vi "Read Raw Log.vi"(5 "Component ID":u8, 7 "FPGA Interface":refnum<class "FPGA Interface.lvclass">, 8 "error in (no error)":errorcluster, 10 "bmReadConfig":T1={"cmdRecordStart"=21632, "cmdRecordLength"=2024, "dataRecordStart"=21632, "dataRecordEnd"=21632} {"dataRecordEnd" format="%04x"; "dataRecordStart" format="%04x"; "cmdRecordStart" format="%04x"}, 11 "48-bit Timetag?":bool) -> (0 "error out":errorcluster, 3 "Raw Log":u16[](array[numeric]) format="%.0x")   [LabVIEW 2016, in "BCI-1553 API.lvlib" / "Bus Monitor.lvclass"]
doc: "Performs the specific reads from the IC to retrieve the entire bus monitor log for a given block of memory. It additionally performs some slight reformatting to the data blocks to get a more easily parsed raw data array."
uses:
  Bus Monitor.lvclass
  Dependencies/FPGA Interface/FPGA Interface.lvclass
  TypeDefs/Bus Monitor Message Type.ctl
  Dependencies/FPGA Interface/rolloverReadConfig.ctl
  TypeDefs/Bus Monitor Read Config.ctl
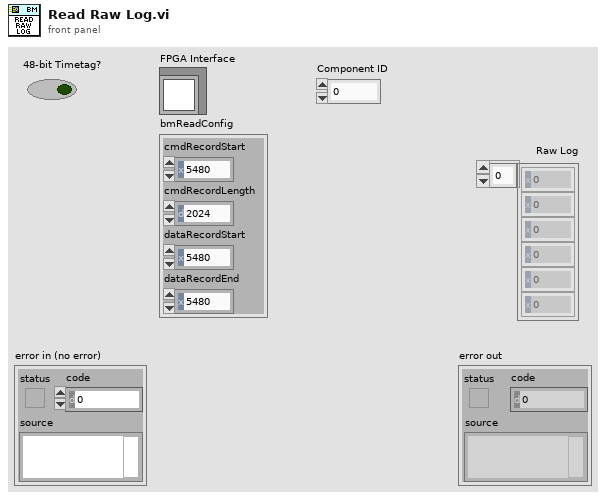
[diagram p1: front panel]
types:
  T1 = typedef "BCI-1553 API.lvlib/Bus Monitor.lvclass/Bus Monitor Read Config.ctl" = cluster{"cmdRecordStart":u16, "cmdRecordLength":u16, "dataRecordStart":u16, "dataRecordEnd":u16}
  T2 = typedef "BCI-1553 API.lvlib/Bus Monitor.lvclass/Bus Monitor Message Type.ctl" = enum16{"Transmit", "Receive", "RT-RT Message", "Mode Code Transmit", "Mode Code Receive", "NULL"}
  T3 = typedef "BCI-1553 API.lvlib/FPGA Interface.lvlib/FPGA Interface.lvclass/rolloverReadConfig.ctl" = cluster{"startAddr":u16, "lowerAddr":u16, "upperAddr":u16}
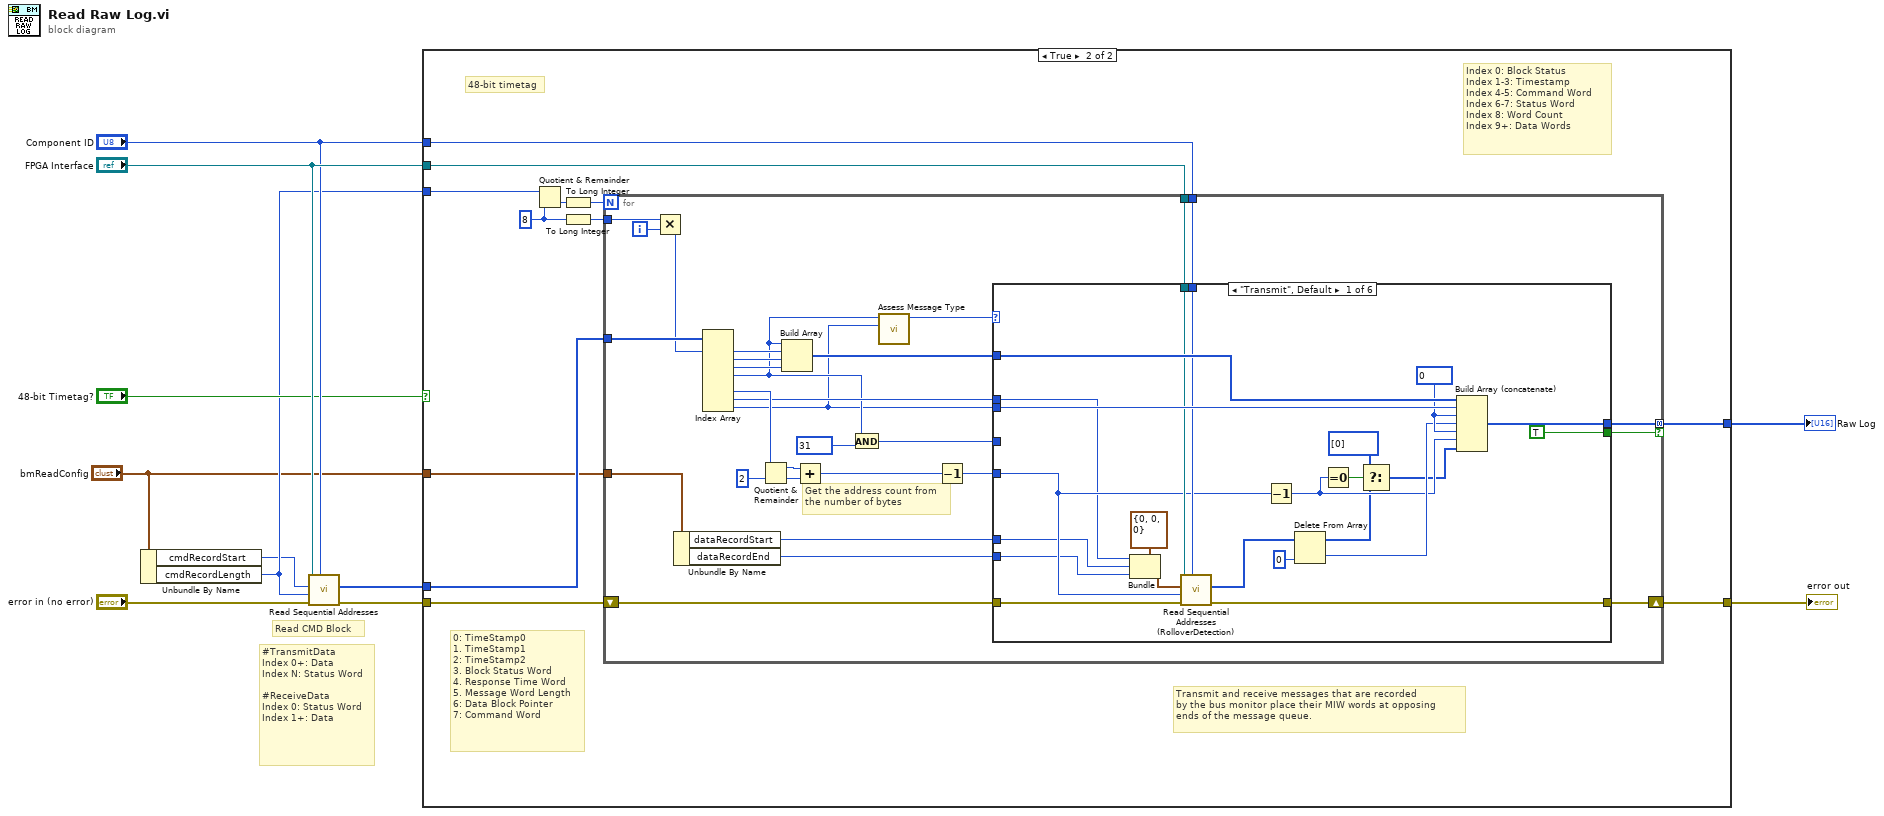
[diagram p0: block diagram]
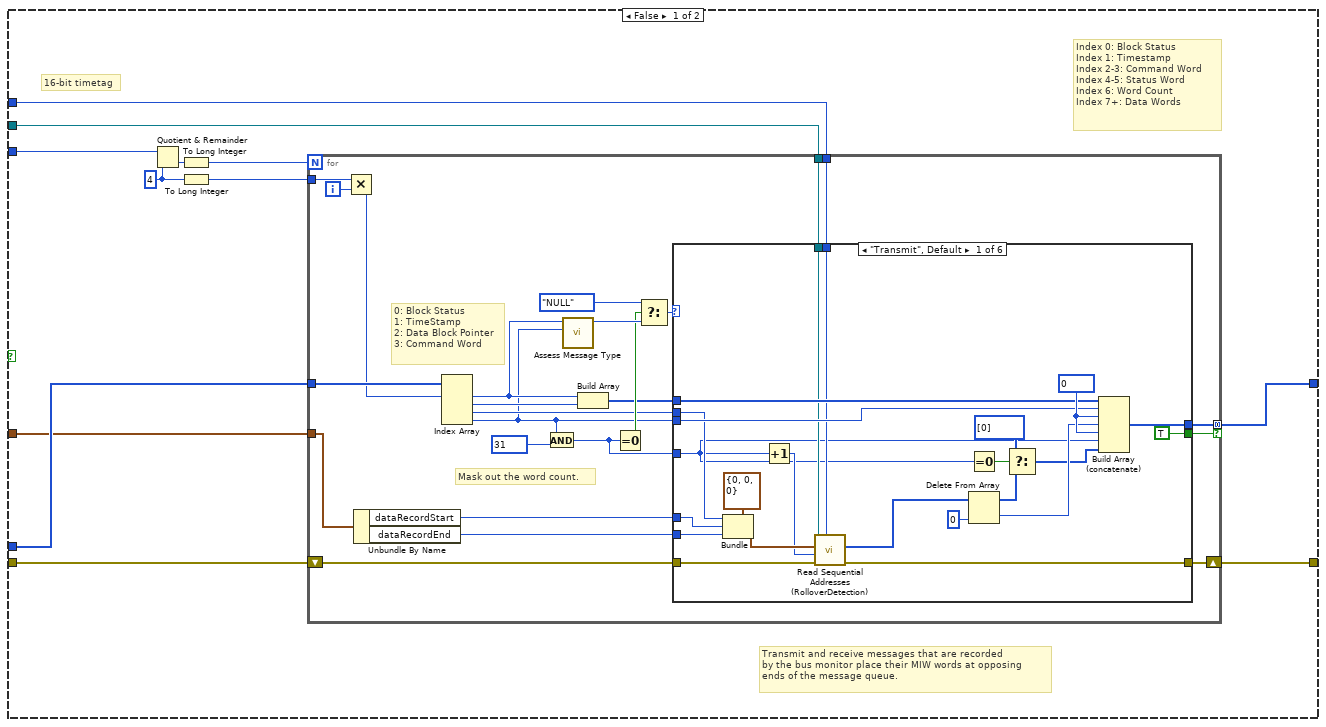
[diagram p2: hidden frame]
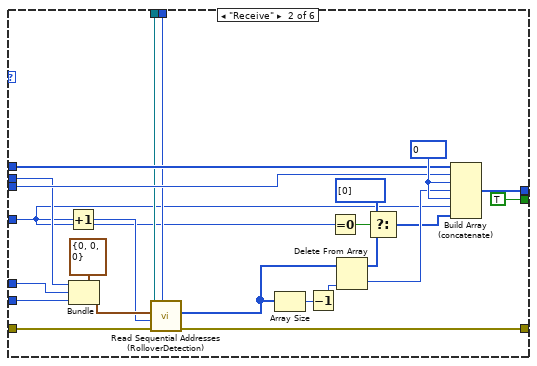
[diagram p3: hidden frame]
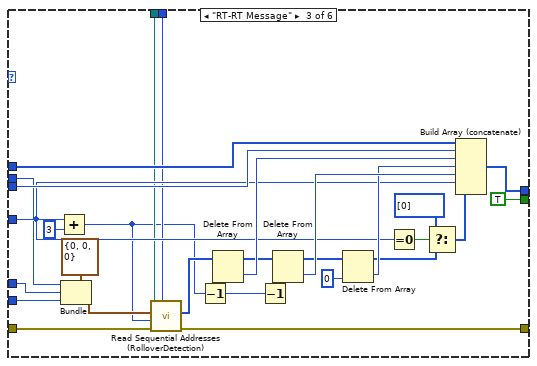
[diagram p4: hidden frame]
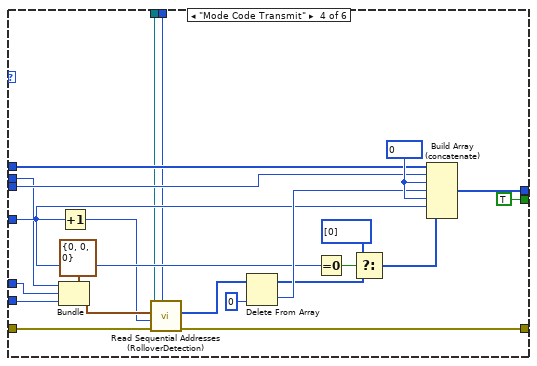
[diagram p5: hidden frame]
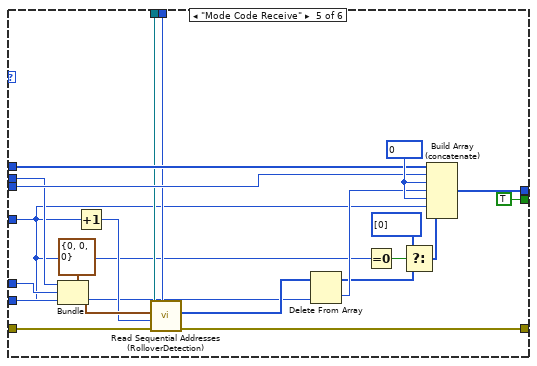
[diagram p6: hidden frame]
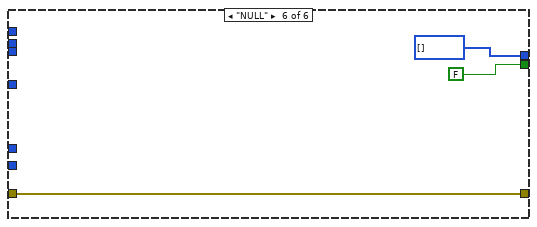
[diagram p7: hidden frame]
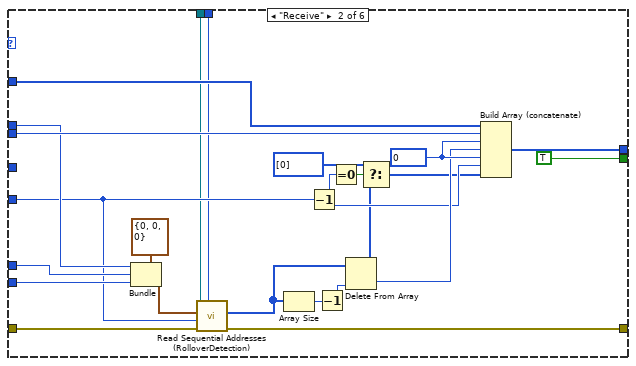
[diagram p8: hidden frame]
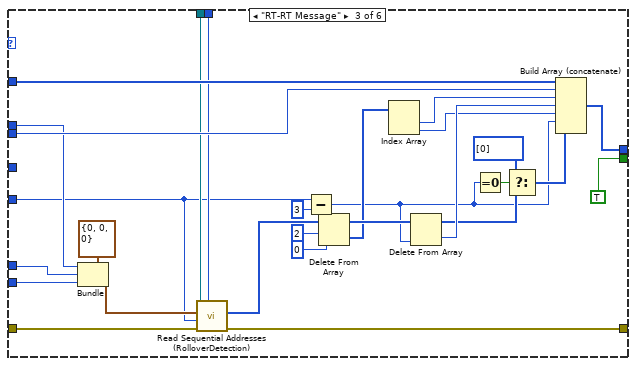
[diagram p9: hidden frame]
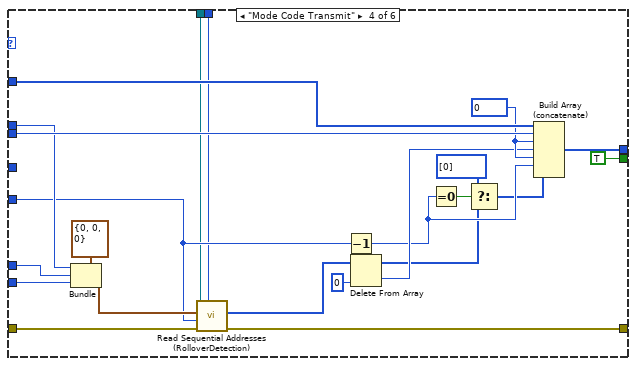
[diagram p10: hidden frame]
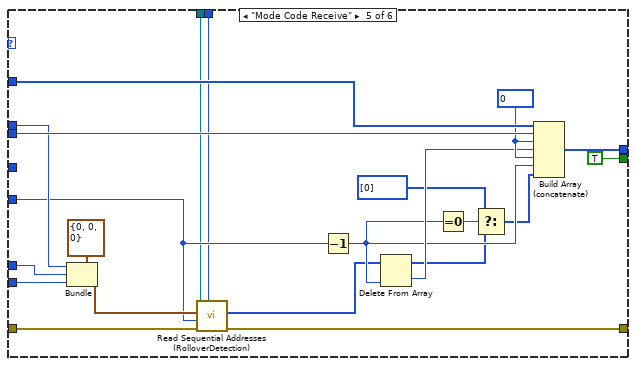
[diagram p11: hidden frame]
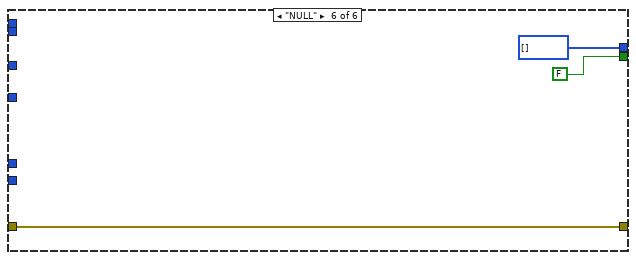
[diagram p12: hidden frame]
diagram:
  # "#TransmitData\nIndex 0+: Data\nIndex N: Status Word\n\n#ReceiveData\nIndex 0: Status Word\nIndex 1+: Data"
  # "Read CMD Block"
  n1 = Unbundle By Name("bmReadConfig") -> ("cmdRecordStart"=w2:u16, "cmdRecordLength"=w3:u16)
  n2 = call-dynamic "Read Sequential Addresses.vi"("Target IC (1-8)"="Component ID", "error in (no error)"="error in (no error)", "Addresses to Read"=w3, "Starting Address"=w2, "FPGA Interface in"="FPGA Interface") -> ("error out"=w11:errorcluster, "Data"=w10:u16[])  [unwired: 5 in]
  n3 = case shown="True" "48-bit Timetag?" {
    tunnel: w11 -> [w23 w183]
    tunnel: w10 -> [w22 w182]
    tunnel: [w18 w178] -> w8
    tunnel: "FPGA Interface" -> [w17 w177]
    tunnel: "Component ID" -> [w16 w176]
    tunnel: w3 -> [w15 w175]
    tunnel: [w14 w174] -> w5
    tunnel: "bmReadConfig" -> [w12 w172]
    frame False {
      w13 = u16 4 ("y")
      # "Index 0: Block Status\nIndex 1: Timestamp\nIndex 2-3: Command Word\nIndex 4-5: Status Word\nIndex 6: Word Count\nIndex 7+: Data Words"
      # "16-bit timetag"
      # "Transmit and receive messages that are recorded\nby the bus monitor place their MIW words at opposing\nends of the message queue."
      n4 = Quotient & Remainder(x=w15, y=w13) -> (floor(x/y)=w21:u16)  [unwired: 1 out]
      n5 = To Long Integer(number=w21) -> (32bit integer=w20:i32)
      n6 = To Long Integer(number=w13) -> (32bit integer=w19:i32)
      n7 = for {
        N: w20 -> [_]
        tunnel: w17 -> [w33]
        tunnel: w16 -> [w32]
        tunnel: w22 -> [w45]
        tunnel: w19 -> [w47]
        tunnel: [w38] -> w14 mode=concatenating if=w37
        shift-right: [w36] -> w18
        shift-left: w23 -> [w39]
        tunnel: w12 -> [w26]
        i -> [w46]
        # "Mask out the word count."
        # "0: Block Status\n1: TimeStamp\n2: Data Block Pointer\n3: Command Word"
        n8 = Multiply(x=w47, y=w46) -> (x*y=w44:i32)
        n9 = Unbundle By Name(w26) -> ("dataRecordStart"=w25:u16, "dataRecordEnd"=w24:u16)
        n10 = Index Array(array=w45, index #1=w44) -> (element #1=w31:u16, element #2=w34:u16, element #3=w28:u16, element #4=w27:u16)  [unwired: 3 in]
        n11 = And(x=w27, y=u16 31 ("Numeric")) -> (x .and. y?=w29:u16)
        n12 = call "Assess Message Type.vi"("Command Word"=w27, "Status Word"=w31) -> ("Message Type"=w42:T2)  [unwired: 9 in]
        n13 = Build Array(w31, w34) -> (w30:u16[])
        n14 = Equal To 0?(x=w29) -> (x = 0?=w40:bool)
        n15 = Select(t=Bus_Monitor_Message_Type."NULL", s=w40, f=w42) -> (s? t:f=w35:T2)
        n16 = case shown="\"Transmit\", Default" w35 {
          tunnel: w39 -> [w55 w78 w103 w132 w156 w171]
          tunnel: [w54 w77 w102 w131 w155 w171] -> w36
          tunnel: w33 -> [w57 w80 w100 w129 w149 _]
          tunnel: w32 -> [w56 w79 w99 w130 w148 _]
          tunnel: [w68 w90 w114 w143 w165 u16[] []] -> w38
          tunnel: [TRUE TRUE TRUE TRUE TRUE FALSE] -> w37
          tunnel: w29 -> [w48 w71 w106 w137 w147 _]
          tunnel: w30 -> [w66 w88 w113 w145 w167 _]
          tunnel: w28 -> [w50 w75 w96 w125 w151 _]
          tunnel: w27 -> [w65 w87 w112 w144 w166 _]
          tunnel: w25 -> [w52 w74 w97 w126 w152 _]
          tunnel: w24 -> [w51 w73 w98 w127 w153 _]
          frame "Transmit", Default {
            w70 = u16 0 ("Numeric")
            n17 = Bundle(cluster=T3 {"startAddr"=0, "lowerAddr"=0, "upperAddr"=0} ("readConfig"), "startAddr"=w50, "lowerAddr"=w52, "upperAddr"=w51) -> (w58:T3)
            n18 = Increment(x=w48) -> (x+1=w49:u16)
            n19 = call-dynamic "Read Sequential Addresses (RolloverDetection).vi"("Target IC (1-8)"=w56, "error in (no error)"=w55, "Addresses to Read"=w49, "readConfig"=w58, "FPGA Interface in"=w57) -> ("error out"=w54:errorcluster, "Data"=w53:u16[])  [unwired: 5 in]
            n20 = Equal To 0?(x=w48) -> (x = 0?=w63:bool)
            n21 = Delete From Array(array=w53, index=0) -> (deleted portion=w69:u16, array with subset deleted=w61:u16[])  [unwired: 1 in]
            n22 = Select(t=u16[] [0] ("Data"), s=w63, f=w61) -> (s? t:f=w60:u16[])
            n23 = Build Array (concatenate)(w66, w65, w70, w69, w70, w48, w60) -> (w68:u16[])
          }
          frame "Receive" {
            w94 = u16 0 ("Numeric")
            n24 = Increment(x=w71) -> (x+1=w72:u16)
            n25 = Bundle(cluster=T3 {"startAddr"=0, "lowerAddr"=0, "upperAddr"=0} ("readConfig"), "startAddr"=w75, "lowerAddr"=w74, "upperAddr"=w73) -> (w81:T3)
            n26 = call-dynamic "Read Sequential Addresses (RolloverDetection).vi"("Target IC (1-8)"=w79, "error in (no error)"=w78, "Addresses to Read"=w72, "readConfig"=w81, "FPGA Interface in"=w80) -> ("error out"=w77:errorcluster, "Data"=w76:u16[])  [unwired: 5 in]
            n27 = Array Size(array=w76) -> (size(s)=w93:i32)
            n28 = Decrement(x=w93) -> (x-1=w91:i32)
            n29 = Equal To 0?(x=w71) -> (x = 0?=w86:bool)
            n30 = Delete From Array(array=w76, index=w91) -> (deleted portion=w92:u16, array with subset deleted=w84:u16[])  [unwired: 1 in]
            n31 = Select(t=u16[] [0] ("Data"), s=w86, f=w84) -> (s? t:f=w83:u16[])
            n32 = Build Array (concatenate)(w88, w87, w94, w92, w94, w71, w83) -> (w90:u16[])
          }
          frame "RT-RT Message" {
            n33 = Add(x=w106, y=u16 3) -> (x+y=w95:u16)
            n34 = Bundle(cluster=T3 {"startAddr"=0, "lowerAddr"=0, "upperAddr"=0} ("readConfig"), "startAddr"=w96, "lowerAddr"=w97, "upperAddr"=w98) -> (w104:T3)
            n35 = call-dynamic "Read Sequential Addresses (RolloverDetection).vi"("Target IC (1-8)"=w99, "error in (no error)"=w103, "Addresses to Read"=w95, "readConfig"=w104, "FPGA Interface in"=w100) -> ("error out"=w102:errorcluster, "Data"=w101:u16[])  [unwired: 5 in]
            n36 = Decrement(x=w95) -> (x-1=w111:u16)
            n37 = Delete From Array(array=w101, index=w111) -> (deleted portion=w122:u16, array with subset deleted=w121:u16[])  [unwired: 1 in]
            n38 = Decrement(x=w111) -> (x-1=w116:u16)
            n39 = Delete From Array(array=w121, index=w116) -> (deleted portion=w120:u16, array with subset deleted=w118:u16[])  [unwired: 1 in]
            n40 = Delete From Array(array=w118, index=0) -> (deleted portion=w117:u16, array with subset deleted=w108:u16[])  [unwired: 1 in]
            n41 = Equal To 0?(x=w106) -> (x = 0?=w110:bool)
            n42 = Select(t=u16[] [0] ("Data"), s=w110, f=w108) -> (s? t:f=w107:u16[])
            n43 = Build Array (concatenate)(w113, w112, w122, w117, w120, w106, w107) -> (w114:u16[])
          }
          frame "Mode Code Transmit" {
            w146 = u16 0 ("Numeric")
            n44 = Bundle(cluster=T3 {"startAddr"=0, "lowerAddr"=0, "upperAddr"=0} ("readConfig"), "startAddr"=w125, "lowerAddr"=w126, "upperAddr"=w127) -> (w133:T3)
            n45 = Increment(x=w137) -> (x+1=w124:u16)
            n46 = call-dynamic "Read Sequential Addresses (RolloverDetection).vi"("Target IC (1-8)"=w130, "error in (no error)"=w132, "Addresses to Read"=w124, "readConfig"=w133, "FPGA Interface in"=w129) -> ("error out"=w131:errorcluster, "Data"=w128:u16[])  [unwired: 5 in]
            n47 = Delete From Array(array=w128, index=0) -> (deleted portion=w140:u16, array with subset deleted=w136:u16[])  [unwired: 1 in]
            n48 = Equal To 0?(x=w137) -> (x = 0?=w139:bool)
            n49 = Select(t=u16[] [0] ("Data"), s=w139, f=w136) -> (s? t:f=w135:u16[])
            n50 = Build Array (concatenate)(w145, w144, w146, w140, w146, w137, w135) -> (w143:u16[])
          }
          frame "Mode Code Receive" {
            w168 = u16 0 ("Numeric")
            n51 = Bundle(cluster=T3 {"startAddr"=0, "lowerAddr"=0, "upperAddr"=0} ("readConfig"), "startAddr"=w151, "lowerAddr"=w152, "upperAddr"=w153) -> (w157:T3)
            n52 = Increment(x=w147) -> (x+1=w150:u16)
            n53 = call-dynamic "Read Sequential Addresses (RolloverDetection).vi"("Target IC (1-8)"=w148, "error in (no error)"=w156, "Addresses to Read"=w150, "readConfig"=w157, "FPGA Interface in"=w149) -> ("error out"=w155:errorcluster, "Data"=w154:u16[])  [unwired: 5 in]
            n54 = Delete From Array(array=w154, index=w147) -> (deleted portion=w163:u16, array with subset deleted=w160:u16[])  [unwired: 1 in]
            n55 = Equal To 0?(x=w147) -> (x = 0?=w162:bool)
            n56 = Select(t=u16[] [0] ("Data"), s=w162, f=w160) -> (s? t:f=w159:u16[])
            n57 = Build Array (concatenate)(w167, w166, w168, w163, w168, w147, w159) -> (w165:u16[])
          }
          frame "NULL" {
          }
        }
      }
    }
    frame True {
      w173 = u16 8 ("y")
      # "Index 0: Block Status\nIndex 1-3: Timestamp\nIndex 4-5: Command Word\nIndex 6-7: Status Word\nIndex 8: Word Count\nIndex 9+: Data Words"
      # "0: TimeStamp0\n1. TimeStamp1\n2: TimeStamp2\n3. Block Status Word\n4. Response Time Word\n5. Message Word Length\n6: Data Block Pointer\n7: Command Word"
      # "48-bit timetag"
      # "Transmit and receive messages that are recorded\nby the bus monitor place their MIW words at opposing\nends of the message queue."
      n58 = Quotient & Remainder(x=w175, y=w173) -> (floor(x/y)=w181:u16)  [unwired: 1 out]
      n59 = To Long Integer(number=w181) -> (32bit integer=w180:i32)
      n60 = To Long Integer(number=w173) -> (32bit integer=w179:i32)
      n61 = for {
        N: w180 -> [_]
        tunnel: w177 -> [w203]
        tunnel: w176 -> [w202]
        tunnel: w182 -> [w210]
        tunnel: w179 -> [w212]
        tunnel: [w198] -> w174 mode=concatenating if=w197
        shift-right: [w204] -> w178
        shift-left: w183 -> [w205]
        tunnel: w172 -> [w186]
        i -> [w211]
        # "Get the address count from\nthe number of bytes"
        n62 = Multiply(x=w212, y=w211) -> (x*y=w209:i32)
        n63 = Unbundle By Name(w186) -> ("dataRecordStart"=w185:u16, "dataRecordEnd"=w184:u16)
        n64 = Index Array(array=w210, index #1=w209) -> (element #1=w201:u16, element #2=w200:u16, element #3=w199:u16, element #4=w191:u16, element #6=w208:u16, element #7=w194:u16, element #8=w190:u16)  [unwired: 7 in, 1 out]
        n65 = Quotient & Remainder(x=w208, y=u16 2) -> (x-y*floor(x/y)=w207:u16, floor(x/y)=w206:u16)
        n66 = Build Array(w191, w201, w200, w199) -> (w193:u16[])
        n67 = Add(x=w207, y=w206) -> (x+y=w188:u16)
        n68 = And(x=w191, y=u16 31 ("Numeric")) -> (x .and. y?=w195:u16)
        n69 = call "Assess Message Type.vi"("Command Word"=w190, "Status Word"=w191) -> ("Message Type"=w189:T2)  [unwired: 9 in]
        n70 = Decrement(x=w188) -> (x-1=w187:u16)
        n71 = case shown="\"Transmit\", Default" w189 {
          tunnel: w205 -> [w219 w238 w265 w293 w316 w335]
          tunnel: [w218 w237 w264 w292 w315 w335] -> w204
          tunnel: w203 -> [w223 w240 w263 w290 w313 _]
          tunnel: w202 -> [w222 w239 w262 w289 w312 _]
          tunnel: [w231 w253 w285 w308 w330 u16[] []] -> w198
          tunnel: [TRUE TRUE TRUE TRUE TRUE FALSE] -> w197
          tunnel: w187 -> [w220 w241 w260 w291 w314 _]
          tunnel: w195 -> [_ _ _ _ _ _]
          tunnel: w194 -> [w216 w244 w268 w294 w317 _]
          tunnel: w193 -> [w235 w259 w287 w309 w331 _]
          tunnel: w190 -> [w234 w258 w286 w307 w329 _]
          tunnel: w185 -> [w215 w243 w267 w296 w318 _]
          tunnel: w184 -> [w214 w242 w266 w295 w319 _]
          frame "Transmit", Default {
            w233 = u16 0 ("Numeric")
            n72 = Bundle(cluster=T3 {"startAddr"=0, "lowerAddr"=0, "upperAddr"=0} ("readConfig"), "startAddr"=w216, "lowerAddr"=w215, "upperAddr"=w214) -> (w213:T3)
            n73 = call-dynamic "Read Sequential Addresses (RolloverDetection).vi"("Target IC (1-8)"=w222, "error in (no error)"=w219, "Addresses to Read"=w220, "readConfig"=w213, "FPGA Interface in"=w223) -> ("error out"=w218:errorcluster, "Data"=w221:u16[])  [unwired: 5 in]
            n74 = Decrement(x=w220) -> (x-1=w226:u16)
            n75 = Delete From Array(array=w221, index=0) -> (deleted portion=w232:u16, array with subset deleted=w225:u16[])  [unwired: 1 in]
            n76 = Equal To 0?(x=w226) -> (x = 0?=w228:bool)
            n77 = Select(t=u16[] [0] ("Data"), s=w228, f=w225) -> (s? t:f=w224:u16[])
            n78 = Build Array (concatenate)(w235, w234, w233, w232, w233, w226, w224) -> (w231:u16[])
          }
          frame "Receive" {
            w257 = u16 0 ("Numeric")
            n79 = Bundle(cluster=T3 {"startAddr"=0, "lowerAddr"=0, "upperAddr"=0} ("readConfig"), "startAddr"=w244, "lowerAddr"=w243, "upperAddr"=w242) -> (w245:T3)
            n80 = call-dynamic "Read Sequential Addresses (RolloverDetection).vi"("Target IC (1-8)"=w239, "error in (no error)"=w238, "Addresses to Read"=w241, "readConfig"=w245, "FPGA Interface in"=w240) -> ("error out"=w237:errorcluster, "Data"=w236:u16[])  [unwired: 5 in]
            n81 = Array Size(array=w236) -> (size(s)=w256:i32)
            n82 = Decrement(x=w241) -> (x-1=w249:u16)
            n83 = Decrement(x=w256) -> (x-1=w254:i32)
            n84 = Equal To 0?(x=w249) -> (x = 0?=w251:bool)
            n85 = Delete From Array(array=w236, index=w254) -> (deleted portion=w255:u16, array with subset deleted=w248:u16[])  [unwired: 1 in]
            n86 = Select(t=u16[] [0] ("Data"), s=w251, f=w248) -> (s? t:f=w247:u16[])
            n87 = Build Array (concatenate)(w259, w258, w257, w255, w257, w249, w247) -> (w253:u16[])
          }
          frame "RT-RT Message" {
            n88 = Bundle(cluster=T3 {"startAddr"=0, "lowerAddr"=0, "upperAddr"=0} ("readConfig"), "startAddr"=w268, "lowerAddr"=w267, "upperAddr"=w266) -> (w269:T3)
            n89 = call-dynamic "Read Sequential Addresses (RolloverDetection).vi"("Target IC (1-8)"=w262, "error in (no error)"=w265, "Addresses to Read"=w260, "readConfig"=w269, "FPGA Interface in"=w263) -> ("error out"=w264:errorcluster, "Data"=w261:u16[])  [unwired: 5 in]
            n90 = Subtract(x=w260, y=u16 3 ("x")) -> (x-y=w271:u16)
            n91 = Delete From Array(array=w261, length=2, index=0) -> (deleted portion=w278:u16[], array with subset deleted=w280:u16[])
            n92 = Index Array(array=w278) -> (element #1=w277:u16, element #2=w276:u16)  [unwired: 2 in]
            n93 = Delete From Array(array=w280, index=w271) -> (deleted portion=w281:u16, array with subset deleted=w273:u16[])  [unwired: 1 in]
            n94 = Equal To 0?(x=w271) -> (x = 0?=w275:bool)
            n95 = Select(t=u16[] [0] ("Data"), s=w275, f=w273) -> (s? t:f=w272:u16[])
            n96 = Build Array (concatenate)(w287, w286, w277, w281, w276, w271, w272) -> (w285:u16[])
          }
          frame "Mode Code Transmit" {
            w306 = u16 0 ("Numeric")
            n97 = Bundle(cluster=T3 {"startAddr"=0, "lowerAddr"=0, "upperAddr"=0} ("readConfig"), "startAddr"=w294, "lowerAddr"=w296, "upperAddr"=w295) -> (w297:T3)
            n98 = call-dynamic "Read Sequential Addresses (RolloverDetection).vi"("Target IC (1-8)"=w289, "error in (no error)"=w293, "Addresses to Read"=w291, "readConfig"=w297, "FPGA Interface in"=w290) -> ("error out"=w292:errorcluster, "Data"=w288:u16[])  [unwired: 5 in]
            n99 = Decrement(x=w291) -> (x-1=w301:u16)
            n100 = Delete From Array(array=w288, index=0) -> (deleted portion=w304:u16, array with subset deleted=w300:u16[])  [unwired: 1 in]
            n101 = Equal To 0?(x=w301) -> (x = 0?=w303:bool)
            n102 = Select(t=u16[] [0] ("Data"), s=w303, f=w300) -> (s? t:f=w299:u16[])
            n103 = Build Array (concatenate)(w309, w307, w306, w304, w306, w301, w299) -> (w308:u16[])
          }
          frame "Mode Code Receive" {
            w328 = u16 0 ("Numeric")
            n104 = Bundle(cluster=T3 {"startAddr"=0, "lowerAddr"=0, "upperAddr"=0} ("readConfig"), "startAddr"=w317, "lowerAddr"=w318, "upperAddr"=w319) -> (w320:T3)
            n105 = call-dynamic "Read Sequential Addresses (RolloverDetection).vi"("Target IC (1-8)"=w312, "error in (no error)"=w316, "Addresses to Read"=w314, "readConfig"=w320, "FPGA Interface in"=w313) -> ("error out"=w315:errorcluster, "Data"=w311:u16[])  [unwired: 5 in]
            n106 = Decrement(x=w314) -> (x-1=w326:u16)
            n107 = Delete From Array(array=w311, index=w326) -> (deleted portion=w327:u16, array with subset deleted=w323:u16[])  [unwired: 1 in]
            n108 = Equal To 0?(x=w326) -> (x = 0?=w325:bool)
            n109 = Select(t=u16[] [0] ("Data"), s=w325, f=w323) -> (s? t:f=w322:u16[])
            n110 = Build Array (concatenate)(w331, w329, w328, w327, w328, w326, w322) -> (w330:u16[])
          }
          frame "NULL" {
          }
        }
      }
    }
  }
  "error out" <- w8
  "Raw Log" <- w5
